vi "Configure Active Apparent Power Low Limit.vi"(0 "VISA resource name":refnum<visa-resource-name>, 5 "Apparent Power Low Limit (40.0)":dbl=40.0 min=0.0 max=500.0 format="%.1f", 11 "error in (no error)":errorcluster) -> (4 "VISA resource name out":refnum<visa-resource-name>, 15 "error out":errorcluster)   [LabVIEW 2016, in "APT 300XAC Series.lvlib"]
doc: "Configures the <B>Frequency Limits</B> of the power source instrument used for testing.\n\n<B>Range</B> : \n310XAC=0.0-1000\n320XAC=0.0-2000\n340XAC=0-4000\n360XAC=0-6000\n\n\nNote : Only supported in Program mode.\n\nThe Apparent Power Low-Limit defines the lower Apparent power limit of the output signal power APT300xAC Series Power Source can reach. Not reaching this value will fail the test\n\nThe Apparent Power High-Limit defines the higher Power limit of the output signal Power APT300xAC Series Power Source can reach. Crossing this value will fail the test"
uses:
  APT 300XAC Series.lvlib
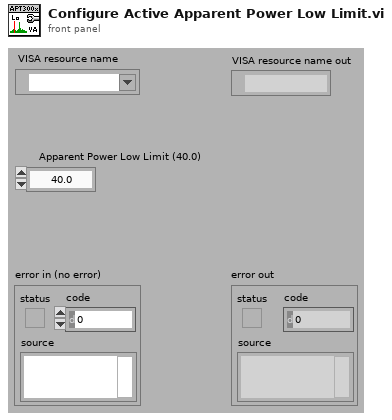
[diagram p1: front panel]
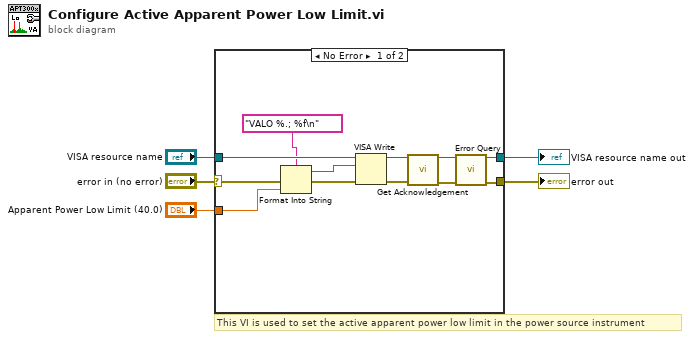
[diagram p0: block diagram]
diagram:
  # "This VI is used to set the active apparent power low limit in the power source instrument"
  n1 = case shown="No Error" "error in (no error)" {
    selector: "error in (no error)" -> [w11 w19]
    tunnel: [w12 w19] -> w5
    tunnel: [w13 w18] -> w4
    tunnel: "VISA resource name" -> [w17 w18]
    tunnel: "Apparent Power Low Limit (40.0)" -> [w16 _]
    frame No Error {
      n2 = Format Into String(format string="VALO %.; %f\n" ("Command"), error in=w11, w16) -> (resulting string=w15:string, error out=w10:errorcluster)  [unwired: 1 in]
      n3 = VISA Write(VISA resource name=w17, write buffer=w15, error in (no error)=w10) -> (VISA resource name out=w7:refnum<visa-resource-name>, error out=w6:errorcluster)  [unwired: 1 out]
      n4 = call "Get Acknowledgement.vi"("VISA resource name"=w7, "error in (no error)"=w6) -> ("VISA resource name out"=w8:refnum<visa-resource-name>, "error out"=w9:errorcluster)  [unwired: 12 in]
      n5 = call "Error Query.vi"("VISA resource name"=w8, "error in (no error)"=w9) -> ("VISA resource name out"=w13:refnum<visa-resource-name>, "error out"=w12:errorcluster)  [unwired: 10 in, 2 out]
    }
    frame Error {
    }
  }
  "error out" <- w5
  "VISA resource name out" <- w4
